vi "Write Export Build Specification.vi"(8 "error in (no error)":errorcluster, 10 "Export Build Specification":path, 11 "Export in":refnum<class "Export.lvclass">) -> (0 "error out":errorcluster, 3 "Export out":refnum<class "Export.lvclass">)   [LabVIEW 2017, in "CL_G3_VIComponentBuilder.lvlib" / "Export.lvclass"]
uses:
  Export.lvclass
  Export.lvclass/Export.ctl
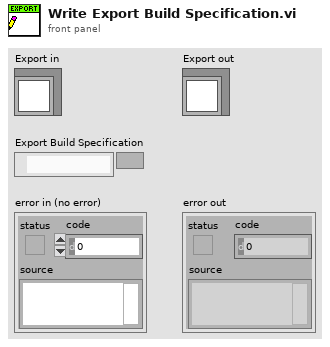
[diagram p1: front panel]
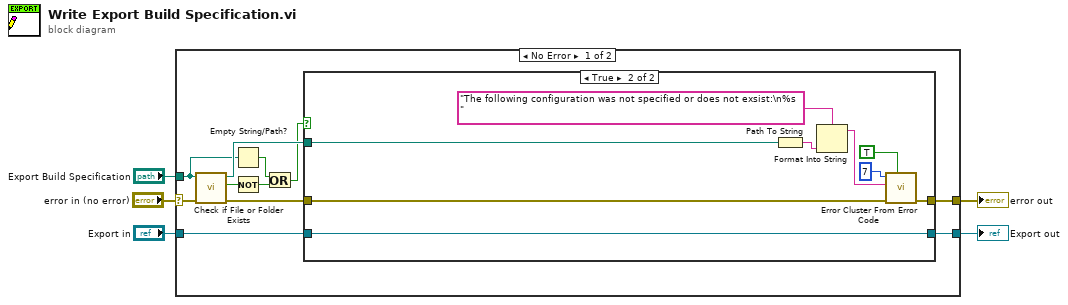
[diagram p0: block diagram]
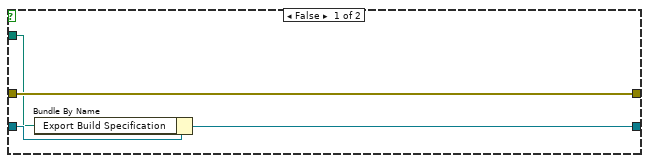
[diagram p2: hidden frame]
diagram:
  n1 = case shown="No Error" "error in (no error)" {
    selector: "error in (no error)" -> [w6 w30]
    tunnel: [w7 w30] -> w4
    tunnel: [w8 w31] -> w2
    tunnel: "Export in" -> [w10 w31]
    tunnel: "Export Build Specification" -> [w9 _]
    frame No Error {
      n2 = call <vilib>:"Check if File or Folder Exists.vi"("error in (no error)"=w6, "path"=w9) -> ("error out"=w15:errorcluster, "file or folder exists?"=w14:bool, "dup path"=w16:path)  [unwired: 7 in]
      n3 = Empty String/Path?(string/path=w9) -> (empty?=w11:bool)
      n4 = Not(x=w14) -> (.not. x?=w13:bool)
      n5 = Or(x=w11, y=w13) -> (x .or. y?=w12:bool)
      n6 = case shown="True" w12 {
        tunnel: [w18 w22] -> w8
        tunnel: w16 -> [w17 w29]
        tunnel: [w20 w21] -> w7
        tunnel: w15 -> [w20 w23]
        tunnel: w10 -> [w19 w22]
        frame False {
          n7 = Bundle By Name(cluster=w19, "Export Build Specification"=w17) -> (w18:refnum<class "Export.lvclass">)
        }
        frame True {
          n8 = Path To String(path=w29) -> (string=w28:string)
          n9 = Format Into String(format string="The following configuration was not specified or does not exsist:\n%s ", w28) -> (resulting string=w24:string)  [unwired: 2 in, 1 out]
          n10 = call <vilib>:"Error Cluster From Error Code.vi"("show call chain? (False)"=TRUE, "error in (no error)"=w23, "error message (\"\")"=w24, "error code (0)"=7) -> ("error out"=w21:errorcluster)  [unwired: 5 in]
        }
      }
    }
    frame Error {
    }
  }
  "error out" <- w4
  "Export out" <- w2
